vi "WriteMessageAttribute.vi"(8 "error in":errorcluster, 9 "attribute":variant, 10 "attribute name":string, 11 "message in":T1) -> (0 "error out":errorcluster, 1 "replaced?":bool, 3 "message out":T1)   [LabVIEW 2013, in "CLM_LocalMessage.lvclass"]
uses:
  CLM_LocalMessage.lvclass
  Message.ctl
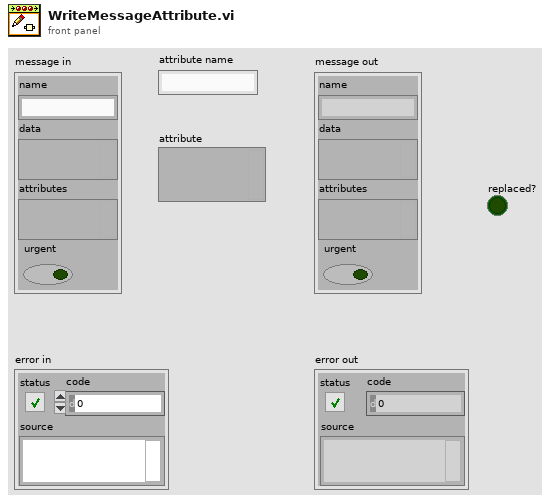
[diagram p1: front panel]
types:
  T1 = typedef "CLM_LocalMessage.lvclass/Message.ctl" = cluster{"name":string, "data":variant, "attributes":variant, "urgent":bool}
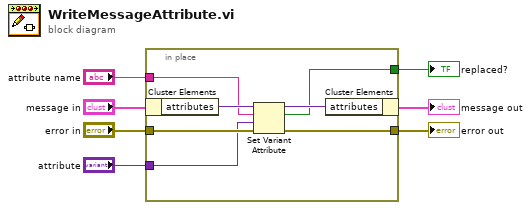
[diagram p0: block diagram]
diagram:
  n1 = in-place {
    in-place-border: "attribute name" -> [w13]
    in-place-border: [w8] -> w4
    in-place-border: "error in" -> [w12]
    in-place-border: [w11] -> w2
    in-place-border: "attribute" -> [w9]
    n2 = in-place-cluster #1("message in") -> ("attributes"=w14:variant)
    n3 = Set Variant Attribute(Variant=w14, name=w13, value=w9, error in=w12) -> (Variant out=w10:variant, replaced=w8:bool, error out=w11:errorcluster)
    n4 = in-place-cluster #1("attributes"=w10) -> (→"message out":T1)
  }
  "replaced?" <- w4
  "error out" <- w2
